vi "rsscope_core_global.vi"() -> ()   [LabVIEW 2014] (continued)
WfmDDNSpectrum1, WfmPNSpectrum1, WfmRNSpectrum1, WfmNBathtub2, WfmNBathMeas2, WfmTNHist2, WfmDNHist2, WfmDDNHist2, WfmPNHist2, WfmRNOHist2, WfmTNTrack2, WfmDDNTrack2, WfmPNTrack2, WfmRNTrack2, WfmTNSpectrum2, WfmDDNSpectrum2, WfmPNSpectrum2, WfmRNSpectrum2, WfmPJDHist1, WfmBUJHist1, WfmRJHist1, WfmPJDTrack1, WfmPJDSpectrum1, WfmPJDHist2, WfmBUJHist2, WfmRJHist2, WfmPJDTrack2, WfmPJDSpectrum2, WfmPNDHist1, WfmBUNHist1, WfmRNHist1, WfmPNDTrack1, WfmPNDSpectrum1, WfmPNDHist2, WfmBUNHist2, WfmRNHist2, WfmPNDTrack2, WfmPNDSpectrum2\r\n\nRemote-control command(s):\nREFLevel<m>:RELative:HYSTeresis"}, {"Level"=2, "Class Only"=TRUE, "Identifier"="", "Descriptive Name"="Tube", "Data Type"=0, "Command"="", "Access"=0, "Range Table"="", "Read Callback"="", "Write Callback"="", "Supported Models"="", "Instrument Options"="", "Flags"=0, "Help"="Configures tube settings for reference levels."}, {"Level"=3, "Class Only"=FALSE, "Identifier"="RSSCOPE_ATTR_TUBE_RELATIVE_OUTER_DISTANCE", "Descriptive Name"="Tube Relative Outer Distance", "Data Type"=1, "Command"="REFL{WfmSuffix}:REL:OTUB", "Access"=2, "Range Table"="RsScope_rngPercent", "Read Callback"="", "Write Callback"="", "Supported Models"="", "Instrument Options"="", "Flags"=0, "Help"="Defines a percentage of the signal level by which the absolute signal level may be larger than the high signal level or lower than the low signal level to be considered high or low, respectively.\n\nAvailable Repeated Capabilities:\nWfmSuffix: WfmNone, WfmC1W1, WfmC1W2, WfmC1W3, WfmC2W1, WfmC2W2, WfmC2W3, WfmC3W1, WfmC3W2, WfmC3W3, WfmC4W1, WfmC4W2, WfmC4W3, WfmMath1, WfmMath2, WfmMath3, WfmMath4, WfmRef1, WfmRef2, WfmRef3, WfmRef4, WfmXY1, WfmXY2, WfmXY3, WfmXY4, WfmMeas1, WfmMeas2, WfmMeas3, WfmMeas4, WfmMeas5, WfmMeas6, WfmMeas7, WfmMeas8, WfmSbus1, WfmSbus2, WfmSbus3, WfmSbus4, WfmD0, WfmD1, WfmD2, WfmD3, WfmD4, WfmD5, WfmD6, WfmD7, WfmD8, WfmD9, WfmD10, WfmD11, WfmD12, WfmD13, WfmD14, WfmD15, WfmMSO1, WfmMSO2, WfmMSO3, WfmMSO4, WfmTRK1, WfmTRK2, WfmTRK3, WfmTRK4, WfmTRK5, WfmTRK6, WfmTRK7, WfmTRK8, WfmSpectrum1, WfmSpectrum2, WfmSpectrum3, WfmSpectrum4, WfmSG1TL1, WfmSG1TL2, WfmSG2TL1, WfmSG2TL2, WfmSG3TL1, WfmSG3TL2, WfmSG4TL1, WfmSG4TL2, WfmEye1, WfmEye2, WfmEye3, WfmEye4, WfmZ1V1, WfmZ1V2, WfmZ1V3, WfmZ1V4, WfmZ1I1, WfmZ1I2, WfmZ1I3, WfmZ1I4, WfmZ2V1, WfmZ2V2, WfmZ2V3, WfmZ2V4, WfmZ2I1, WfmZ2I2, WfmZ2I3, WfmZ2I4, WfmDiff1, WfmDiff2, WfmCommon1, WfmCommon2, WfmTDRZ, WfmTDRH, WfmTDRR, WfmMath5, WfmMath6, WfmMath7, WfmMath8, WfmSpectrum5, WfmSpectrum6, WfmSpectrum7, WfmSpectrum8, WfmSG5TL1, WfmSG5TL2, WfmSG6TL1, WfmSG6TL2, WfmSG7TL1, WfmSG7TL2, WfmSG8TL1, WfmSG8TL2, WfmHP1, WfmHP2, WfmHP3, WfmHP4, WfmHP5, WfmHP6, WfmHP7, WfmHP8, WfmHP9, WfmHP10, WfmBathtub1, WfmBathMeas1, WfmStepResp1, WfmSRHist1, WfmSDHist1, WfmTJHist1, WfmDJHist1, WfmDDJHist1, WfmPJHist1, WfmRJOHist1, WfmSRTrack1, WfmTJTrack1, WfmDJTrack1, WfmDDJTrack1, WfmPJTrack1, WfmRJTrack1, WfmTJSpectrum1, WfmDDJSpectrum1, WfmPJSpectrum1, WfmRJSpectrum1, WfmSEye1, WfmBathtub2, WfmBathMeas2, WfmStepResp2, WfmSRHist2, WfmSDHist2, WfmTJHist2, WfmDJHist2, WfmDDJHist2, WfmPJHist2, WfmRJOHist2, WfmSRTrack2, WfmSDTrack2, WfmTJTrack2, WfmDDJTrack2, WfmPJTrack2, WfmRJTrack2, WfmTJSpectrum2, WfmDDJSpectrum2, WfmPJSpectrum2, WfmRJSpectrum2, WfmSEye2, WfmNBathtub1, WfmNBathMeas1, WfmTNHist1, WfmDNHist1, WfmDDNHist1, WfmPNHist1, WfmRNOTrack1, WfmTNTrack1, WfmDDNTrack1, WfmPNTrack1, WfmRNTrack1, WfmTNSpectrum1, WfmDDNSpectrum1, WfmPNSpectrum1, WfmRNSpectrum1, WfmNBathtub2, WfmNBathMeas2, WfmTNHist2, WfmDNHist2, WfmDDNHist2, WfmPNHist2, WfmRNOHist2, WfmTNTrack2, WfmDDNTrack2, WfmPNTrack2, WfmRNTrack2, WfmTNSpectrum2, WfmDDNSpectrum2, WfmPNSpectrum2, WfmRNSpectrum2, WfmPJDHist1, WfmBUJHist1, WfmRJHist1, WfmPJDTrack1, WfmPJDSpectrum1, WfmPJDHist2, WfmBUJHist2, WfmRJHist2, WfmPJDTrack2, WfmPJDSpectrum2, WfmPNDHist1, WfmBUNHist1, WfmRNHist1, WfmPNDTrack1, WfmPNDSpectrum1, WfmPNDHist2, WfmBUNHist2, WfmRNHist2, WfmPNDTrack2, WfmPNDSpectrum2\r\n\nRemote-control command(s):\nREFLevel<m>:RELative:OTUBe"}, {"Level"=3, "Class Only"=FALSE, "Identifier"="RSSCOPE_ATTR_TUBE_RELATIVE_INNER_DISTANCE", "Descriptive Name"="Tube Relative Inner Distance", "Data Type"=1, "Command"="REFL{WfmSuffix}:REL:ITUB", "Access"=2, "Range Table"="RsScope_rngTubeRelativeInnerDistance", "Read Callback"="", "Write Callback"="", "Supported Models"="", "Instrument Options"="", "Flags"=0, "Help"="Defines a percentage of the signal level by which the absolute signal level may be higher than the low signal level or lower than the high signal level to be considered low or high, respectively.\n\nAvailable Repeated Capabilities:\nWfmSuffix: WfmNone, WfmC1W1, WfmC1W2, WfmC1W3, WfmC2W1, WfmC2W2, WfmC2W3, WfmC3W1, WfmC3W2, WfmC3W3, WfmC4W1, WfmC4W2, WfmC4W3, WfmMath1, WfmMath2, WfmMath3, WfmMath4, WfmRef1, WfmRef2, WfmRef3, WfmRef4, WfmXY1, WfmXY2, WfmXY3, WfmXY4, WfmMeas1, WfmMeas2, WfmMeas3, WfmMeas4, WfmMeas5, WfmMeas6, WfmMeas7, WfmMeas8, WfmSbus1, WfmSbus2, WfmSbus3, WfmSbus4, WfmD0, WfmD1, WfmD2, WfmD3, WfmD4, WfmD5, WfmD6, WfmD7, WfmD8, WfmD9, WfmD10, WfmD11, WfmD12, WfmD13, WfmD14, WfmD15, WfmMSO1, WfmMSO2, WfmMSO3, WfmMSO4, WfmTRK1, WfmTRK2, WfmTRK3, WfmTRK4, WfmTRK5, WfmTRK6, WfmTRK7, WfmTRK8, WfmSpectrum1, WfmSpectrum2, WfmSpectrum3, WfmSpectrum4, WfmSG1TL1, WfmSG1TL2, WfmSG2TL1, WfmSG2TL2, WfmSG3TL1, WfmSG3TL2, WfmSG4TL1, WfmSG4TL2, WfmEye1, WfmEye2, WfmEye3, WfmEye4, WfmZ1V1, WfmZ1V2, WfmZ1V3, WfmZ1V4, WfmZ1I1, WfmZ1I2, WfmZ1I3, WfmZ1I4, WfmZ2V1, WfmZ2V2, WfmZ2V3, WfmZ2V4, WfmZ2I1, WfmZ2I2, WfmZ2I3, WfmZ2I4, WfmDiff1, WfmDiff2, WfmCommon1, WfmCommon2, WfmTDRZ, WfmTDRH, WfmTDRR, WfmMath5, WfmMath6, WfmMath7, WfmMath8, WfmSpectrum5, WfmSpectrum6, WfmSpectrum7, WfmSpectrum8, WfmSG5TL1, WfmSG5TL2, WfmSG6TL1, WfmSG6TL2, WfmSG7TL1, WfmSG7TL2, WfmSG8TL1, WfmSG8TL2, WfmHP1, WfmHP2, WfmHP3, WfmHP4, WfmHP5, WfmHP6, WfmHP7, WfmHP8, WfmHP9, WfmHP10, WfmBathtub1, WfmBathMeas1, WfmStepResp1, WfmSRHist1, WfmSDHist1, WfmTJHist1, WfmDJHist1, WfmDDJHist1, WfmPJHist1, WfmRJOHist1, WfmSRTrack1, WfmTJTrack1, WfmDJTrack1, WfmDDJTrack1, WfmPJTrack1, WfmRJTrack1, WfmTJSpectrum1, WfmDDJSpectrum1, WfmPJSpectrum1, WfmRJSpectrum1, WfmSEye1, WfmBathtub2, WfmBathMeas2, WfmStepResp2, WfmSRHist2, WfmSDHist2, WfmTJHist2, WfmDJHist2, WfmDDJHist2, WfmPJHist2, WfmRJOHist2, WfmSRTrack2, WfmSDTrack2, WfmTJTrack2, WfmDDJTrack2, WfmPJTrack2, WfmRJTrack2, WfmTJSpectrum2, WfmDDJSpectrum2, WfmPJSpectrum2, WfmRJSpectrum2, WfmSEye2, WfmNBathtub1, WfmNBathMeas1, WfmTNHist1, WfmDNHist1, WfmDDNHist1, WfmPNHist1, WfmRNOTrack1, WfmTNTrack1, WfmDDNTrack1, WfmPNTrack1, WfmRNTrack1, WfmTNSpectrum1, WfmDDNSpectrum1, WfmPNSpectrum1, WfmRNSpectrum1, WfmNBathtub2, WfmNBathMeas2, WfmTNHist2, WfmDNHist2, WfmDDNHist2, WfmPNHist2, WfmRNOHist2, WfmTNTrack2, WfmDDNTrack2, WfmPNTrack2, WfmRNTrack2, WfmTNSpectrum2, WfmDDNSpectrum2, WfmPNSpectrum2, WfmRNSpectrum2, WfmPJDHist1, WfmBUJHist1, WfmRJHist1, WfmPJDTrack1, WfmPJDSpectrum1, WfmPJDHist2, WfmBUJHist2, WfmRJHist2, WfmPJDTrack2, WfmPJDSpectrum2, WfmPNDHist1, WfmBUNHist1, WfmRNHist1, WfmPNDTrack1, WfmPNDSpectrum1, WfmPNDHist2, WfmBUNHist2, WfmRNHist2, WfmPNDTrack2, WfmPNDSpectrum2\r\n\nRemote-control command(s):\nREFLevel<m>:RELative:ITUBe"}, {"Level"=3, "Class Only"=FALSE, "Identifier"="RSSCOPE_ATTR_TUBE_ABSOLUTE_TOP_OUTER_DISTANCE", "Descriptive Name"="Tube Absolute Top Outer Distance", "Data Type"=1, "Command"="REFL{WfmSuffix}:ABS:TOT", "Access"=2, "Range Table"="", "Read Callback"="", "Write Callback"="", "Supported Models"="", "Instrument Options"="", "Flags"=0, "Help"="Defines an area above the high signal level which is still considered to be high level.\n\nAvailable Repeated Capabilities:\nWfmSuffix: WfmNone, WfmC1W1, WfmC1W2, WfmC1W3, WfmC2W1, WfmC2W2, WfmC2W3, WfmC3W1, WfmC3W2, WfmC3W3, WfmC4W1, WfmC4W2, WfmC4W3, WfmMath1, WfmMath2, WfmMath3, WfmMath4, WfmRef1, WfmRef2, WfmRef3, WfmRef4, WfmXY1, WfmXY2, WfmXY3, WfmXY4, WfmMeas1, WfmMeas2, WfmMeas3, WfmMeas4, WfmMeas5, WfmMeas6, WfmMeas7, WfmMeas8, WfmSbus1, WfmSbus2, WfmSbus3, WfmSbus4, WfmD0, WfmD1, WfmD2, WfmD3, WfmD4, WfmD5, WfmD6, WfmD7, WfmD8, WfmD9, WfmD10, WfmD11, WfmD12, WfmD13, WfmD14, WfmD15, WfmMSO1, WfmMSO2, WfmMSO3, WfmMSO4, WfmTRK1, WfmTRK2, WfmTRK3, WfmTRK4, WfmTRK5, WfmTRK6, WfmTRK7, WfmTRK8, WfmSpectrum1, WfmSpectrum2, WfmSpectrum3, WfmSpectrum4, WfmSG1TL1, WfmSG1TL2, WfmSG2TL1, WfmSG2TL2, WfmSG3TL1, WfmSG3TL2, WfmSG4TL1, WfmSG4TL2, WfmEye1, WfmEye2, WfmEye3, WfmEye4, WfmZ1V1, WfmZ1V2, WfmZ1V3, WfmZ1V4, WfmZ1I1, WfmZ1I2, WfmZ1I3, WfmZ1I4, WfmZ2V1, WfmZ2V2, WfmZ2V3, WfmZ2V4, WfmZ2I1, WfmZ2I2, WfmZ2I3, WfmZ2I4, WfmDiff1, WfmDiff2, WfmCommon1, WfmCommon2, WfmTDRZ, WfmTDRH, WfmTDRR, WfmMath5, WfmMath6, WfmMath7, WfmMath8, WfmSpectrum5, WfmSpectrum6, WfmSpectrum7, WfmSpectrum8, WfmSG5TL1, WfmSG5TL2, WfmSG6TL1, WfmSG6TL2, WfmSG7TL1, WfmSG7TL2, WfmSG8TL1, WfmSG8TL2, WfmHP1, WfmHP2, WfmHP3, WfmHP4, WfmHP5, WfmHP6, WfmHP7, WfmHP8, WfmHP9, WfmHP10, WfmBathtub1, WfmBathMeas1, WfmStepResp1, WfmSRHist1, WfmSDHist1, WfmTJHist1, WfmDJHist1, WfmDDJHist1, WfmPJHist1, WfmRJOHist1, WfmSRTrack1, WfmTJTrack1, WfmDJTrack1, WfmDDJTrack1, WfmPJTrack1, WfmRJTrack1, WfmTJSpectrum1, WfmDDJSpectrum1, WfmPJSpectrum1, WfmRJSpectrum1, WfmSEye1, WfmBathtub2, WfmBathMeas2, WfmStepResp2, WfmSRHist2, WfmSDHist2, WfmTJHist2, WfmDJHist2, WfmDDJHist2, WfmPJHist2, WfmRJOHist2, WfmSRTrack2, WfmSDTrack2, WfmTJTrack2, WfmDDJTrack2, WfmPJTrack2, WfmRJTrack2, WfmTJSpectrum2, WfmDDJSpectrum2, WfmPJSpectrum2, WfmRJSpectrum2, WfmSEye2, WfmNBathtub1, WfmNBathMeas1, WfmTNHist1, WfmDNHist1, WfmDDNHist1, WfmPNHist1, WfmRNOTrack1, WfmTNTrack1, WfmDDNTrack1, WfmPNTrack1, WfmRNTrack1, WfmTNSpectrum1, WfmDDNSpectrum1, WfmPNSpectrum1, WfmRNSpectrum1, WfmNBathtub2, WfmNBathMeas2, WfmTNHist2, WfmDNHist2, WfmDDNHist2, WfmPNHist2, WfmRNOHist2, WfmTNTrack2, WfmDDNTrack2, WfmPNTrack2, WfmRNTrack2, WfmTNSpectrum2, WfmDDNSpectrum2, WfmPNSpectrum2, WfmRNSpectrum2, WfmPJDHist1, WfmBUJHist1, WfmRJHist1, WfmPJDTrack1, WfmPJDSpectrum1, WfmPJDHist2, WfmBUJHist2, WfmRJHist2, WfmPJDTrack2, WfmPJDSpectrum2, WfmPNDHist1, WfmBUNHist1, WfmRNHist1, WfmPNDTrack1, WfmPNDSpectrum1, WfmPNDHist2, WfmBUNHist2, WfmRNHist2, WfmPNDTrack2, WfmPNDSpectrum2\r\n\nRemote-control command(s):\nREFLevel<m>:ABSolute:TOTube"}, {"Level"=3, "Class Only"=FALSE, "Identifier"="RSSCOPE_ATTR_TUBE_ABSOLUTE_TOP_INNER_DISTANCE", "Descriptive Name"="Tube Absolute Top Inner Distance", "Data Type"=1, "Command"="REFL{WfmSuffix}:ABS:TIT", "Access"=2, "Range Table"="", "Read Callback"="", "Write Callback"="", "Supported Models"="", "Instrument Options"="", "Flags"=0, "Help"="Defines an area beneath the high signal level which is still considered to be high level.\n\nAvailable Repeated Capabilities:\nWfmSuffix: WfmNone, WfmC1W1, WfmC1W2, WfmC1W3, WfmC2W1, WfmC2W2, WfmC2W3, WfmC3W1, WfmC3W2, WfmC3W3, WfmC4W1, WfmC4W2, WfmC4W3, WfmMath1, WfmMath2, WfmMath3, WfmMath4, WfmRef1, WfmRef2, WfmRef3, WfmRef4, WfmXY1, WfmXY2, WfmXY3, WfmXY4, WfmMeas1, WfmMeas2, WfmMeas3, WfmMeas4, WfmMeas5, WfmMeas6, WfmMeas7, WfmMeas8, WfmSbus1, WfmSbus2, WfmSbus3, WfmSbus4, WfmD0, WfmD1, WfmD2, WfmD3, WfmD4, WfmD5, WfmD6, WfmD7, WfmD8, WfmD9, WfmD10, WfmD11, WfmD12, WfmD13, WfmD14, WfmD15, WfmMSO1, WfmMSO2, WfmMSO3, WfmMSO4, WfmTRK1, WfmTRK2, WfmTRK3, WfmTRK4, WfmTRK5, WfmTRK6, WfmTRK7, WfmTRK8, WfmSpectrum1, WfmSpectrum2, WfmSpectrum3, WfmSpectrum4, WfmSG1TL1, WfmSG1TL2, WfmSG2TL1, WfmSG2TL2, WfmSG3TL1, WfmSG3TL2, WfmSG4TL1, WfmSG4TL2, WfmEye1, WfmEye2, WfmEye3, WfmEye4, WfmZ1V1, WfmZ1V2, WfmZ1V3, WfmZ1V4, WfmZ1I1, WfmZ1I2, WfmZ1I3, WfmZ1I4, WfmZ2V1, WfmZ2V2, WfmZ2V3, WfmZ2V4, WfmZ2I1, WfmZ2I2, WfmZ2I3, WfmZ2I4, WfmDiff1, WfmDiff2, WfmCommon1, WfmCommon2, WfmTDRZ, WfmTDRH, WfmTDRR, WfmMath5, WfmMath6, WfmMath7, WfmMath8, WfmSpectrum5, WfmSpectrum6, WfmSpectrum7, WfmSpectrum8, WfmSG5TL1, WfmSG5TL2, WfmSG6TL1, WfmSG6TL2, WfmSG7TL1, WfmSG7TL2, WfmSG8TL1, WfmSG8TL2, WfmHP1, WfmHP2, WfmHP3, WfmHP4, WfmHP5, WfmHP6, WfmHP7, WfmHP8, WfmHP9, WfmHP10, WfmBathtub1, WfmBathMeas1, WfmStepResp1, WfmSRHist1, WfmSDHist1, WfmTJHist1, WfmDJHist1, WfmDDJHist1, WfmPJHist1, WfmRJOHist1, WfmSRTrack1, WfmTJTrack1, WfmDJTrack1, WfmDDJTrack1, WfmPJTrack1, WfmRJTrack1, WfmTJSpectrum1, WfmDDJSpectrum1, WfmPJSpectrum1, WfmRJSpectrum1, WfmSEye1, WfmBathtub2, WfmBathMeas2, WfmStepResp2, WfmSRHist2, WfmSDHist2, WfmTJHist2, WfmDJHist2, WfmDDJHist2, WfmPJHist2, WfmRJOHist2, WfmSRTrack2, WfmSDTrack2, WfmTJTrack2, WfmDDJTrack2, WfmPJTrack2, WfmRJTrack2, WfmTJSpectrum2, WfmDDJSpectrum2, WfmPJSpectrum2, WfmRJSpectrum2, WfmSEye2, WfmNBathtub1, WfmNBathMeas1, WfmTNHist1, WfmDNHist1, WfmDDNHist1, WfmPNHist1, WfmRNOTrack1, WfmTNTrack1, WfmDDNTrack1, WfmPNTrack1, WfmRNTrack1, WfmTNSpectrum1, WfmDDNSpectrum1, WfmPNSpectrum1, WfmRNSpectrum1, WfmNBathtub2, WfmNBathMeas2, WfmTNHist2, WfmDNHist2, WfmDDNHist2, WfmPNHist2, WfmRNOHist2, WfmTNTrack2, WfmDDNTrack2, WfmPNTrack2, WfmRNTrack2, WfmTNSpectrum2, WfmDDNSpectrum2, WfmPNSpectrum2, WfmRNSpectrum2, WfmPJDHist1, WfmBUJHist1, WfmRJHist1, WfmPJDTrack1, WfmPJDSpectrum1, WfmPJDHist2, WfmBUJHist2, WfmRJHist2, WfmPJDTrack2, WfmPJDSpectrum2, WfmPNDHist1, WfmBUNHist1, WfmRNHist1, WfmPNDTrack1, WfmPNDSpectrum1, WfmPNDHist2, WfmBUNHist2, WfmRNHist2, WfmPNDTrack2, WfmPNDSpectrum2\r\n\nRemote-control command(s):\nREFLevel<m>:ABSolute:TITube"}, {"Level"=3, "Class Only"=FALSE, "Identifier"="RSSCOPE_ATTR_TUBE_ABSOLUTE_BOTTOM_INNER_DISTANCE", "Descriptive Name"="Tube Absolute Bottom Inner Distance", "Data Type"=1, "Command"="REFL{WfmSuffix}:ABS:BIT", "Access"=2, "Range Table"="", "Read Callback"="", "Write Callback"="", "Supported Models"="", "Instrument Options"="", "Flags"=0, "Help"="Defines an area above the low signal level which is still considered to be low level.\n\nAvailable Repeated Capabilities:\nWfmSuffix: WfmNone, WfmC1W1, WfmC1W2, WfmC1W3, WfmC2W1, WfmC2W2, WfmC2W3, WfmC3W1, WfmC3W2, WfmC3W3, WfmC4W1, WfmC4W2, WfmC4W3, WfmMath1, WfmMath2, WfmMath3, WfmMath4, WfmRef1, WfmRef2, WfmRef3, WfmRef4, WfmXY1, WfmXY2, WfmXY3, WfmXY4, WfmMeas1, WfmMeas2, WfmMeas3, WfmMeas4, WfmMeas5, WfmMeas6, WfmMeas7, WfmMeas8, WfmSbus1, WfmSbus2, WfmSbus3, WfmSbus4, WfmD0, WfmD1, WfmD2, WfmD3, WfmD4, WfmD5, WfmD6, WfmD7, WfmD8, WfmD9, WfmD10, WfmD11, WfmD12, WfmD13, WfmD14, WfmD15, WfmMSO1, WfmMSO2, WfmMSO3, WfmMSO4, WfmTRK1, WfmTRK2, WfmTRK3, WfmTRK4, WfmTRK5, WfmTRK6, WfmTRK7, WfmTRK8, WfmSpectrum1, WfmSpectrum2, WfmSpectrum3, WfmSpectrum4, WfmSG1TL1, WfmSG1TL2, WfmSG2TL1, WfmSG2TL2, WfmSG3TL1, WfmSG3TL2, WfmSG4TL1, WfmSG4TL2, WfmEye1, WfmEye2, WfmEye3, WfmEye4, WfmZ1V1, WfmZ1V2, WfmZ1V3, WfmZ1V4, WfmZ1I1, WfmZ1I2, WfmZ1I3, WfmZ1I4, WfmZ2V1, WfmZ2V2, WfmZ2V3, WfmZ2V4, WfmZ2I1, WfmZ2I2, WfmZ2I3, WfmZ2I4, WfmDiff1, WfmDiff2, WfmCommon1, WfmCommon2, WfmTDRZ, WfmTDRH, WfmTDRR, WfmMath5, WfmMath6, WfmMath7, WfmMath8, WfmSpectrum5, WfmSpectrum6, WfmSpectrum7, WfmSpectrum8, WfmSG5TL1, WfmSG5TL2, WfmSG6TL1, WfmSG6TL2, WfmSG7TL1, WfmSG7TL2, WfmSG8TL1, WfmSG8TL2, WfmHP1, WfmHP2, WfmHP3, WfmHP4, WfmHP5, WfmHP6, WfmHP7, WfmHP8, WfmHP9, WfmHP10, WfmBathtub1, WfmBathMeas1, WfmStepResp1, WfmSRHist1, WfmSDHist1, WfmTJHist1, WfmDJHist1, WfmDDJHist1, WfmPJHist1, WfmRJOHist1, WfmSRTrack1, WfmTJTrack1, WfmDJTrack1, WfmDDJTrack1, WfmPJTrack1, WfmRJTrack1, WfmTJSpectrum1, WfmDDJSpectrum1, WfmPJSpectrum1, WfmRJSpectrum1, WfmSEye1, WfmBathtub2, WfmBathMeas2, WfmStepResp2, WfmSRHist2, WfmSDHist2, WfmTJHist2, WfmDJHist2, WfmDDJHist2, WfmPJHist2, WfmRJOHist2, WfmSRTrack2, WfmSDTrack2, WfmTJTrack2, WfmDDJTrack2, WfmPJTrack2, WfmRJTrack2, WfmTJSpectrum2, WfmDDJSpectrum2, WfmPJSpectrum2, WfmRJSpectrum2, WfmSEye2, WfmNBathtub1, WfmNBathMeas1, WfmTNHist1, WfmDNHist1, WfmDDNHist1, WfmPNHist1, WfmRNOTrack1, WfmTNTrack1, WfmDDNTrack1, WfmPNTrack1, WfmRNTrack1, WfmTNSpectrum1, WfmDDNSpectrum1, WfmPNSpectrum1, WfmRNSpectrum1, WfmNBathtub2, WfmNBathMeas2, WfmTNHist2, WfmDNHist2, WfmDDNHist2, WfmPNHist2, WfmRNOHist2, WfmTNTrack2, WfmDDNTrack2, WfmPNTrack2, WfmRNTrack2, WfmTNSpectrum2, WfmDDNSpectrum2, WfmPNSpectrum2, WfmRNSpectrum2, WfmPJDHist1, WfmBUJHist1, WfmRJHist1, WfmPJDTrack1, WfmPJDSpectrum1, WfmPJDHist2, WfmBUJHist2, WfmRJHist2, WfmPJDTrack2, WfmPJDSpectrum2, WfmPNDHist1, WfmBUNHist1, WfmRNHist1, WfmPNDTrack1, WfmPNDSpectrum1, WfmPNDHist2, WfmBUNHist2, WfmRNHist2, WfmPNDTrack2, WfmPNDSpectrum2\r\n\nRemote-control command(s):\nREFLevel<m>:ABSolute:BITube"}, {"Level"=3, "Class Only"=FALSE, "Identifier"="RSSCOPE_ATTR_TUBE_ABSOLUTE_BOTTOM_OUTER_DISTANCE", "Descriptive Name"="Tube Absolute Bottom Outer Distance", "Data Type"=1, "Command"="REFL{WfmSuffix}:ABS:BOT", "Access"=2, "Range Table"="", "Read Callback"="", "Write Callback"="", "Supported Models"="", "Instrument Options"="", "Flags"=0, "Help"="Defines an area beneath the low signal level which is still considered to be low level.\n\nAvailable Repeated Capabilities:\nWfmSuffix: WfmNone, WfmC1W1, WfmC1W2, WfmC1W3, WfmC2W1, WfmC2W2, WfmC2W3, WfmC3W1, WfmC3W2, WfmC3W3, WfmC4W1, WfmC4W2, WfmC4W3, WfmMath1, WfmMath2, WfmMath3, WfmMath4, WfmRef1, WfmRef2, WfmRef3, WfmRef4, WfmXY1, WfmXY2, WfmXY3, WfmXY4, WfmMeas1, WfmMeas2, WfmMeas3, WfmMeas4, WfmMeas5, WfmMeas6, WfmMeas7, WfmMeas8, WfmSbus1, WfmSbus2, WfmSbus3, WfmSbus4, WfmD0, WfmD1, WfmD2, WfmD3, WfmD4, WfmD5, WfmD6, WfmD7, WfmD8, WfmD9, WfmD10, WfmD11, WfmD12, WfmD13, WfmD14, WfmD15, WfmMSO1, WfmMSO2, WfmMSO3, WfmMSO4, WfmTRK1, WfmTRK2, WfmTRK3, WfmTRK4, WfmTRK5, WfmTRK6, WfmTRK7, WfmTRK8, WfmSpectrum1, WfmSpectrum2, WfmSpectrum3, WfmSpectrum4, WfmSG1TL1, WfmSG1TL2, WfmSG2TL1, WfmSG2TL2, WfmSG3TL1, WfmSG3TL2, WfmSG4TL1, WfmSG4TL2, WfmEye1, WfmEye2, WfmEye3, WfmEye4, WfmZ1V1, WfmZ1V2, WfmZ1V3, WfmZ1V4, WfmZ1I1, WfmZ1I2, WfmZ1I3, WfmZ1I4, WfmZ2V1, WfmZ2V2, WfmZ2V3, WfmZ2V4, WfmZ2I1, WfmZ2I2, WfmZ2I3, WfmZ2I4, WfmDiff1, WfmDiff2, WfmCommon1, WfmCommon2, WfmTDRZ, WfmTDRH, WfmTDRR, WfmMath5, WfmMath6, WfmMath7, WfmMath8, WfmSpectrum5, WfmSpectrum6, WfmSpectrum7, WfmSpectrum8, WfmSG5TL1, WfmSG5TL2, WfmSG6TL1, WfmSG6TL2, WfmSG7TL1, WfmSG7TL2, WfmSG8TL1, WfmSG8TL2, WfmHP1, WfmHP2, WfmHP3, WfmHP4, WfmHP5, WfmHP6, WfmHP7, WfmHP8, WfmHP9, WfmHP10, WfmBathtub1, WfmBathMeas1, WfmStepResp1, WfmSRHist1, WfmSDHist1, WfmTJHist1, WfmDJHist1, WfmDDJHist1, WfmPJHist1, WfmRJOHist1, WfmSRTrack1, WfmTJTrack1, WfmDJTrack1, WfmDDJTrack1, WfmPJTrack1, WfmRJTrack1, WfmTJSpectrum1, WfmDDJSpectrum1, WfmPJSpectrum1, WfmRJSpectrum1, WfmSEye1, WfmBathtub2, WfmBathMeas2, WfmStepResp2, WfmSRHist2, WfmSDHist2, WfmTJHist2, WfmDJHist2, WfmDDJHist2, WfmPJHist2, WfmRJOHist2, WfmSRTrack2, WfmSDTrack2, WfmTJTrack2, WfmDDJTrack2, WfmPJTrack2, WfmRJTrack2, WfmTJSpectrum2, WfmDDJSpectrum2, WfmPJSpectrum2, WfmRJSpectrum2, WfmSEye2, WfmNBathtub1, WfmNBathMeas1, WfmTNHist1, WfmDNHist1, WfmDDNHist1, WfmPNHist1, WfmRNOTrack1, WfmTNTrack1, WfmDDNTrack1, WfmPNTrack1, WfmRNTrack1, WfmTNSpectrum1, WfmDDNSpectrum1, WfmPNSpectrum1, WfmRNSpectrum1, WfmNBathtub2, WfmNBathMeas2, WfmTNHist2, WfmDNHist2, WfmDDNHist2, WfmPNHist2, WfmRNOHist2, WfmTNTrack2, WfmDDNTrack2, WfmPNTrack2, WfmRNTrack2, WfmTNSpectrum2, WfmDDNSpectrum2, WfmPNSpectrum2, WfmRNSpectrum2, WfmPJDHist1, WfmBUJHist1, WfmRJHist1, WfmPJDTrack1, WfmPJDSpectrum1, WfmPJDHist2, WfmBUJHist2, WfmRJHist2, WfmPJDTrack2, WfmPJDSpectrum2, WfmPNDHist1, WfmBUNHist1, WfmRNHist1, WfmPNDTrack1, WfmPNDSpectrum1, WfmPNDHist2, WfmBUNHist2, WfmRNHist2, WfmPNDTrack2, WfmPNDSpectrum2\r\n\nRemote-control command(s):\nREFLevel<m>:ABSolute:BOTube"}, {"Level"=1, "Class Only"=TRUE, "Identifier"="", "Descriptive Name"="Mathematics", "Data Type"=0, "Command"="", "Access"=0, "Range Table"="", "Read Callback"="", "Write Callback"="", "Supported Models"="", "Instrument Options"="", "Flags"=0, "Help"="The R&S RTO provides different methods of creating mathematical waveforms:\n- Applying mathematical functions to source data\n- Performing FFT analysis on source data"}, {"Level"=2, "Class Only"=TRUE, "Identifier"="", "Descriptive Name"="General Mathematics", "Data Type"=0, "Command"="", "Access"=0, "Range Table"="", "Read Callback"="", "Write Callback"="", "Supported Models"="", "Instrument Options"="", "Flags"=0, "Help"="General mathematics parameters."}, {"Level"=3, "Class Only"=FALSE, "Identifier"="RSSCOPE_ATTR_MATH_WAVEFORM_ENABLED", "Descriptive Name"="Math Waveform Enabled", "Data Type"=3, "Command"="CALC:MATH{Math}:STAT", "Access"=2, "Range Table"="", "Read Callback"="", "Write Callback"="", "Supported Models"="", "Instrument Options"="", "Flags"=0, "Help"="Enables the math waveform display.\n\nAvailable Repeated Capabilities:\nMath: M1, M2, M3, M4, M5, M6, M7, M8\r\n\nRemote-control command(s):\nCALCulate:MATH<m>:STATe"}, {"Level"=3, "Class Only"=FALSE, "Identifier"="RSSCOPE_ATTR_MATH_WAVEFORM_ENVELOPE_SELECTION", "Descriptive Name"="Math Envelope Selection", "Data Type"=0, "Command"="CALC:MATH{Math}:ENVS", "Access"=2, "Range Table"="rsscope_rngWaveformSelection", "Read Callback"="", "Write Callback"="", "Supported Models"="", "Instrument Options"="", "Flags"=0, "Help"="Selects the upper or lower part of the waveform for mathematic calculation, or a combination of both.\n\nThe setting is relevant for waveforms with waveform arithmetic mode &apos;Envelope&apos; or with &apos;Peak detect&apos; decimation. All mathematic operations - except for derivation - can be applied to envelope waveforms and waveforms with &apos;Peak detect&apos; decimation.\n\nAvailable Repeated Capabilities:\nMath: M1, M2, M3, M4, M5, M6, M7, M8\r\n\nRemote-control command(s):\nCALCulate:MATH<m>:ENVSelection"}, {"Level"=3, "Class Only"=FALSE, "Identifier"="RSSCOPE_ATTR_MATH_ACQUISITION_TYPE", "Descriptive Name"="Math Acquisition Type", "Data Type"=0, "Command"="CALC:MATH{Math}:ARIT", "Access"=2, "Range Table"="rsscope_rngWaveformArithmetics", "Read Callback"="", "Write Callback"="", "Supported Models"="", "Instrument Options"="", "Flags"=0, "Help"="Selects the method to build the resulting math waveform from consecutive acquisitions. The processing is similar to the waveform arithmetics - instead of the acquired waveforms the math waveforms are used to create envelope and average.\n\nAvailable Repeated Capabilities:\nMath: M1, M2, M3, M4, M5, M6, M7, M8\r\n\nRemote-control command(s):\nCALCulate:MATH<m>:ARIThmetics"}, {"Level"=3, "Class Only"=FALSE, "Identifier"="RSSCOPE_ATTR_MATH_EXPRESSION", "Descriptive Name"="Math Expression", "Data Type"=2, "Command"="CALC:MATH{Math}", "Access"=2, "Range Table"="", "Read Callback"="", "Write Callback"="", "Supported Models"="", "Instrument Options"="", "Flags"=0, "Help"="Defines the math expression to be calculated for the specified math channel.\n\nAvailable Repeated Capabilities:\nMath: M1, M2, M3, M4, M5, M6, M7, M8\r\n\nRemote-control command(s):\nCALCulate:MATH<m>[:EXPRession][:DEFine]"}, {"Level"=3, "Class Only"=FALSE, "Identifier"="RSSCOPE_ATTR_MATH_VERTICAL_RANGE", "Descriptive Name"="Math Vertical Range", "Data Type"=1, "Command"="CALC:MATH{Math}:VERT:RANG", "Access"=2, "Range Table"="RsScope_rngMathVerticalRange", "Read Callback"="", "Write Callback"="", "Supported Models"="", "Instrument Options"="", "Flags"=0, "Help"="Defines the range of FFT values to be displayed.\n\nAvailable Repeated Capabilities:\nMath: M1, M2, M3, M4, M5, M6, M7, M8\r\n\nRemote-control command(s):\nCALCulate:MATH<m>:VERTical:RANGe"}, {"Level"=3, "Class Only"=FALSE, "Identifier"="RSSCOPE_ATTR_MATH_VERTICAL_SCALE", "Descriptive Name"="Math Vertical Scale", "Data Type"=1, "Command"="CALC:MATH{Math}:VERT:SCAL", "Access"=2, "Range Table"="rsscope_rngMathVerticalScale", "Read Callback"="", "Write Callback"="", "Supported Models"="", "Instrument Options"="", "Flags"=0, "Help"="Defines the scale of the y-axis in the math function diagram. The value is defined as &apos;V per division&apos;, e.g. 50V/div. In this case, the horizontal grid lines are displayed in intervals of 50 V.\n\nAvailable Repeated Capabilities:\nMath: M1, M2, M3, M4, M5, M6, M7, M8\r\n\nRemote-control command(s):\nCALCulate:MATH<m>:VERTical:SCALe"}, {"Level"=3, "Class Only"=FALSE, "Identifier"="RSSCOPE_ATTR_MATH_VERTICAL_OFFSET", "Descriptive Name"="Math Vertical Offset", "Data Type"=1, "Command"="CALC:MATH{Math}:VERT:OFFS", "Access"=2, "Range Table"="RsScope_rngMathVerticalOffset", "Read Callback"="", "Write Callback"="", "Supported Models"="", "Instrument Options"="", "Flags"=0, "Help"="Sets a voltage offset to adjust the vertical position of the math function on the screen.\n\nAvailable Repeated Capabilities:\nMath: M1, M2, M3, M4, M5, M6, M7, M8\r\n\nRemote-control command(s):\nCALCulate:MATH<m>:VERTical:OFFSet"}, {"Level"=3, "Class Only"=FALSE, "Identifier"="RSSCOPE_ATTR_MATH_RESET", "Descriptive Name"="Math Reset", "Data Type"=4, "Command"="ACQ:ARES:IMM", "Access"=1, "Range Table"="", "Read Callback"="", "Write Callback"="", "Supported Models"="", "Instrument Options"="", "Flags"=0, "Help"="Forces the immediate restart of the envelope and average calculation for all waveforms.\n\nAvailable Repeated Capabilities:\nNone\n\nRemote-control command(s):\nACQuire:ARESet:IMMediate"}, {"Level"=3, "Class Only"=FALSE, "Identifier"="RSSCOPE_ATTR_MATH_RESET_MODE", "Descriptive Name"="Math Reset Mode", "Data Type"=0, "Command"="ACQ:ARES:MODE", "Access"=2, "Range Table"="rsscope_rngMathResetMode", "Read Callback"="", "Write Callback"="", "Supported Models"="", "Instrument Options"="", "Flags"=0, "Help"="Defines when the envelope and average evaluation restarts.\n\nAvailable Repeated Capabilities:\nNone\n\nRemote-control command(s):\nACQuire:ARESet:MODE"}, {"Level"=3, "Class Only"=FALSE, "Identifier"="RSSCOPE_ATTR_MATH_ENVELOPE_TIMEOUT", "Descriptive Name"="Math Envelope Timeout", "Data Type"=1, "Command"="ACQ:ARES:TIME", "Access"=2, "Range Table"="rsscope_rngMathEnvelopeTime", "Read Callback"="", "Write Callback"="", "Supported Models"="", "Instrument Options"="", "Flags"=0, "Help"="Defines the time after which the envelope and average evaluation restarts.\n\nAvailable Repeated Capabilities:\nNone\n\nRemote-control command(s):\nACQuire:ARESet:TIME"}, {"Level"=3, "Class Only"=FALSE, "Identifier"="RSSCOPE_ATTR_MATH_ACQUIRED_WAVEFORMS", "Descriptive Name"="Math Acquired Waveforms", "Data Type"=0, "Command"="ACQ:ARES:COUN", "Access"=2, "Range Table"="rsscope_rngMathAcquiredWaveforms", "Read Callback"="", "Write Callback"="", "Supported Models"="", "Instrument Options"="", "Flags"=0, "Help"="Defines the number of acquired waveforms after which the envelope and average evaluation restarts.\n\nAvailable Repeated Capabilities:\nNone\n\nRemote-control command(s):\nACQuire:ARESet:COUNt"}, {"Level"=2, "Class Only"=TRUE, "Identifier"="", "Descriptive Name"="FFT", "Data Type"=0, "Command"="", "Access"=0, "Range Table"="", "Read Callback"="", "Write Callback"="", "Supported Models"="", "Instrument Options"="", "Flags"=0, "Help"="Attributes for setting FFT parameters. During FFT analysis, a signal in the time domain is  converted to a spectrum of frequencies. A basic FFT waveform can be displayed very quickly. By defining additional FFT parameters, the waveform can be configured in more detail. As a result, either the magnitude or the phase of the determined frequencies can be displayed, or more complex FFT functions. Analysis can be restricted to an extract of the original time base, and the results display can be restricted to a specified frequency range."}, {"Level"=3, "Class Only"=FALSE, "Identifier"="RSSCOPE_ATTR_FFT_TYPE", "Descriptive Name"="FFT Type", "Data Type"=0, "Command"="CALC:MATH{Math}:FFT:TYPE", "Access"=2, "Range Table"="RsScope_rngFFTType", "Read Callback"="", "Write Callback"="", "Supported Models"="", "Instrument Options"="", "Flags"=0, "Help"="Selects between the magnitude and phase spectrum type.\n\nAvailable Repeated Capabilities:\nMath: M1, M2, M3, M4, M5, M6, M7, M8\r\n\nRemote-control command(s):\nCALCulate:MATH<m>:FFT:TYPE"}, {"Level"=3, "Class Only"=FALSE, "Identifier"="RSSCOPE_ATTR_FFT_FREQUENCY_AXIS", "Descriptive Name"="FFT Frequency Axis", "Data Type"=0, "Command"="CALC:MATH{Math}:FFT:LOGS", "Access"=2, "Range Table"="RsScope_rngLinLog", "Read Callback"="", "Write Callback"="", "Supported Models"="", "Instrument Options"="", "Flags"=0, "Help"="Defines the scaling method for the frequency (x-)axis of the spectrogram.\n\nAvailable Repeated Capabilities:\nMath: M1, M2, M3, M4, M5, M6, M7, M8\r\n\nRemote-control command(s):\nCALCulate:MATH<m>:FFT:LOGScale"}, {"Level"=3, "Class Only"=FALSE, "Identifier"="RSSCOPE_ATTR_FFT_CENTER_FREQUENCY", "Descriptive Name"="FFT Center Frequency", "Data Type"=1, "Command"="CALC:MATH{Math}:FFT:CFR", "Access"=2, "Range Table"="", "Read Callback"="", "Write Callback"="", "Supported Models"="", "Instrument Options"="", "Flags"=0, "Help"="Defines the position of the displayed frequency range, which is (Center - Span/2) to (Center + Span/2).\n\nAvailable Repeated Capabilities:\nMath: M1, M2, M3, M4, M5, M6, M7, M8\r\n\nRemote-control command(s):\nCALCulate:MATH<m>:FFT:CFRequency"}, {"Level"=3, "Class Only"=FALSE, "Identifier"="RSSCOPE_ATTR_FFT_FREQUENCY_SPAN", "Descriptive Name"="FFT Frequency Span", "Data Type"=1, "Command"="CALC:MATH{Math}:FFT:SPAN", "Access"=2, "Range Table"="", "Read Callback"="", "Write Callback"="", "Supported Models"="", "Instrument Options"="", "Flags"=0, "Help"="The span is specified in Hertz and defines the width of the displayed frequency range, which is (Center - Span/2) to (Center + Span/2).\n\nAvailable Repeated Capabilities:\nMath: M1, M2, M3, M4, M5, M6, M7, M8\r\n\nRemote-control command(s):\nCALCulate:MATH<m>:FFT:SPAN"}, {"Level"=3, "Class Only"=FALSE, "Identifier"="RSSCOPE_ATTR_FFT_FULL_SPAN", "Descriptive Name"="FFT Full Span", "Data Type"=4, "Command"="CALC:MATH{Math}:FFT:FULL", "Access"=1, "Range Table"="", "Read Callback"="", "Write Callback"="", "Supported Models"="", "Instrument Options"="", "Flags"=0, "Help"="Performs FFT calculation for the full frequency span.\n\nAvailable Repeated Capabilities:\nMath: M1, M2, M3, M4, M5, M6, M7, M8\r\n\nRemote-control command(s):\nCALCulate:MATH<m>:FFT:FULLspan"}, {"Level"=3, "Class Only"=FALSE, "Identifier"="RSSCOPE_ATTR_FFT_START_FREQUENCY", "Descriptive Name"="FFT Start Frequency", "Data Type"=1, "Command"="CALC:MATH{Math}:FFT:STAR", "Access"=2, "Range Table"="", "Read Callback"="", "Write Callback"="", "Supported Models"="", "Instrument Options"="", "Flags"=0, "Help"="Defines the start frequency of the displayed frequency span.\n\nAvailable Repeated Capabilities:\nMath: M1, M2, M3, M4, M5, M6, M7, M8\r\n\nRemote-control command(s):\nCALCulate:MATH<m>:FFT:STARt"}, {"Level"=3, "Class Only"=FALSE, "Identifier"="RSSCOPE_ATTR_FFT_STOP_FREQUENCY", "Descriptive Name"="FFT Stop Frequency", "Data Type"=1, "Command"="CALC:MATH{Math}:FFT:STOP", "Access"=2, "Range Table"="", "Read Callback"="", "Write Callback"="", "Supported Models"="", "Instrument Options"="", "Flags"=0, "Help"="Defines the stop frequency of the displayed frequency span.\n\nAvailable Repeated Capabilities:\nMath: M1, M2, M3, M4, M5, M6, M7, M8\r\n\nRemote-control command(s):\nCALCulate:MATH<m>:FFT:STOP"}, {"Level"=3, "Class Only"=FALSE, "Identifier"="RSSCOPE_ATTR_FFT_WINDOW_TYPE", "Descriptive Name"="FFT Window Type", "Data Type"=0, "Command"="CALC:MATH{Math}:FFT:WIND:TYPE", "Access"=2, "Range Table"="rsscope_rngFFTWindowType", "Read Callback"="", "Write Callback"="", "Supported Models"="", "Instrument Options"="", "Flags"=0, "Help"="Windowing helps minimize the discontinuities at the end of the measured signal interval and thus reduces the effect of spectral leakage, increasing the frequency resolution.\nVarious different window functions are provided in the R&S RTO to suit different input signals. Each of the window functions has specific characteristics, including some advantages and some trade-offs. These characteristics need to be considered carefully to find the optimum solution for the measurement task.\n\nAvailable Repeated Capabilities:\nMath: M1, M2, M3, M4, M5, M6, M7, M8\r\n\nRemote-control command(s):\nCALCulate:MATH<m>:FFT:WINDow:TYPE"}, {"Level"=3, "Class Only"=FALSE, "Identifier"="RSSCOPE_ATTR_FFT_USE_COLOR_TABLE", "Descriptive Name"="FFT Use Color Table", "Data Type"=3, "Command"="CALC:MATH{Math}:FFT:USEC", "Access"=2, "Range Table"="", "Read Callback"="", "Write Callback"="", "Supported Models"="", "Instrument Options"="", "Flags"=0, "Help"="If enabled, the selected waveform is displayed according to its assigned color table.\n\nAvailable Repeated Capabilities:\nMath: M1, M2, M3, M4, M5, M6, M7, M8\r\n\nRemote-control command(s):\nCALCulate:MATH<m>:FFT:USEColtab"}, {"Level"=3, "Class Only"=FALSE, "Identifier"="RSSCOPE_ATTR_FFT_REFERENCE_LEVEL", "Descriptive Name"="FFT Reference Level", "Data Type"=1, "Command"="CALC:MATH{Math}:FFT:MAGN:LEV", "Access"=2, "Range Table"="rsscope_rngFFTReferenceLevel", "Read Callback"="", "Write Callback"="", "Supported Models"="", "Instrument Options"="", "Flags"=0, "Help"="Defines the reference level for dB scaling.\n\nAvailable Repeated Capabilities:\nMath: M1, M2, M3, M4, M5, M6, M7, M8\r\n\nRemote-control command(s):\nCALCulate:MATH<m>:FFT:MAGNitude:LEVel"}, {"Level"=3, "Class Only"=FALSE, "Identifier"="RSSCOPE_ATTR_FFT_MAGNITUDE_RANGE", "Descriptive Name"="FFT Magnitude Range", "Data Type"=0, "Command"="CALC:MATH{Math}:FFT:MAGN:RANG", "Access"=2, "Range Table"="rsscope_rngFFTRange", "Read Callback"="", "Write Callback"="", "Supported Models"="", "Instrument Options"="", "Flags"=0, "Help"="Defines the vertical value range in spectrum mode.\n\nAvailable Repeated Capabilities:\nMath: M1, M2, M3, M4, M5, M6, M7, M8\r\n\nRemote-control command(s):\nCALCulate:MATH<m>:FFT:MAGNitude:RANGe"}, {"Level"=3, "Class Only"=FALSE, "Identifier"="RSSCOPE_ATTR_FFT_MAGNITUDE_UNIT", "Descriptive Name"="FFT Magnitude Unit", "Data Type"=0, "Command"="CALC:MATH{Math}:FFT:MAGN:SCAL", "Access"=2, "Range Table"="rsscope_rngFFTMagnitudeUnit", "Read Callback"="", "Write Callback"="", "Supported Models"="", "Instrument Options"="", "Flags"=0, "Help"="Defines the scaling of the y-axis. The display values are valid for 50Ohm termination impendance.\n\nAvailable Repeated Capabilities:\nMath: M1, M2, M3, M4, M5, M6, M7, M8\r\n\nRemote-control command(s):\nCALCulate:MATH<m>:FFT:MAGNitude:SCALe"}, {"Level"=3, "Class Only"=FALSE, "Identifier"="RSSCOPE_ATTR_FFT_PHASE_UNIT", "Descriptive Name"="FFT Phase Unit", "Data Type"=0, "Command"="CALC:MATH{Math}:FFT:PHAS:SCAL", "Access"=2, "Range Table"="rsscope_rngFFTPhaseUnit", "Read Callback"="", "Write Callback"="", "Supported Models"="", "Instrument Options"="", "Flags"=0, "Help"="Defines the scaling unit for phase display.\n\nAvailable Repeated Capabilities:\nMath: M1, M2, M3, M4, M5, M6, M7, M8\r\n\nRemote-control command(s):\nCALCulate:MATH<m>:FFT:PHASe:SCALe"}, {"Level"=3, "Class Only"=FALSE, "Identifier"="RSSCOPE_ATTR_FFT_PHASE_UNWRAP_ENABLED", "Descriptive Name"="FFT Phase Unwrap Enabled", "Data Type"=3, "Command"="CALC:MATH{Math}:FFT:PHAS:UNWR", "Access"=2, "Range Table"="", "Read Callback"="", "Write Callback"="", "Supported Models"="", "Instrument Options"="", "Flags"=0, "Help"="If enabled, phase shifts due to a limitation of the value range are eliminated.\n\nAvailable Repeated Capabilities:\nMath: M1, M2, M3, M4, M5, M6, M7, M8\r\n\nRemote-control command(s):\nCALCulate:MATH<m>:FFT:PHASe:UNWRap"}, {"Level"=3, "Class Only"=FALSE, "Identifier"="RSSCOPE_ATTR_FFT_NOISE_SUPPRESSION_ENABLED", "Descriptive Name"="FFT Noise Suppression Enabled", "Data Type"=3, "Command"="CALC:MATH{Math}:FFT:PHAS:SUPP", "Access"=2, "Range Table"="", "Read Callback"="", "Write Callback"="", "Supported Models"="", "Instrument Options"="", "Flags"=0, "Help"="Enables noise suppression.\n\nAvailable Repeated Capabilities:\nMath: M1, M2, M3, M4, M5, M6, M7, M8\r\n\nRemote-control command(s):\nCALCulate:MATH<m>:FFT:PHASe:SUPPression"}, {"Level"=3, "Class Only"=FALSE, "Identifier"="RSSCOPE_ATTR_FFT_NOISE_SUPPRESSION_THRESHOLD", "Descriptive Name"="FFT Noise Suppression Threshold", "Data Type"=1, "Command"="CALC:MATH{Math}:FFT:PHAS:THR", "Access"=2, "Range Table"="rsscope_rngSuppressionThreshold", "Read Callback"="", "Write Callback"="", "Supported Models"="", "Instrument Options"="", "Flags"=0, "Help"="Defines the minimum frequency magnitude for which phases are calculated.\n\nAvailable Repeated Capabilities:\nMath: M1, M2, M3, M4, M5, M6, M7, M8\r\n\nRemote-control command(s):\nCALCulate:MATH<m>:FFT:PHASe:THReshold"}, {"Level"=3, "Class Only"=FALSE, "Identifier"="RSSCOPE_ATTR_FFT_VERTICAL_MAXIMUM", "Descriptive Name"="FFT Vertical Maximum", "Data Type"=1, "Command"="CALC:MATH{Math}:VERT:MAX", "Access"=2, "Range Table"="RsScope_rngFFTVerticalMaximum", "Read Callback"="", "Write Callback"="", "Supported Models"="", "Instrument Options"="", "Flags"=0, "Help"="Defines the maximum value on y-axis for spectrum displays.\n\nAvailable Repeated Capabilities:\nMath: M1, M2, M3, M4, M5, M6, M7, M8\r\n\nRemote-control command(s):\nCALCulate:MATH<m>:VERTical:MAXimum"}, {"Level"=3, "Class Only"=FALSE, "Identifier"="RSSCOPE_ATTR_FFT_RESOLUTION_BANDWIDTH", "Descriptive Name"="FFT Resolution Bandwidth", "Data Type"=1, "Command"="CALC:MATH{Math}:FFT:BAND", "Access"=2, "Range Table"="rsscope_rngRBW", "Read Callback"="", "Write Callback"="", "Supported Models"="", "Instrument Options"="", "Flags"=0, "Help"="Defines the resolution bandwidth.\n\nAvailable Repeated Capabilities:\nMath: M1, M2, M3, M4, M5, M6, M7, M8\r\n\nRemote-control command(s):\nCALCulate:MATH<m>:FFT:BANDwidth[:RESolution][:VALue]"}, {"Level"=3, "Class Only"=FALSE, "Identifier"="RSSCOPE_ATTR_FFT_RESOLUTION_BANDWIDTH_COUPLING_ENABLED", "Descriptive Name"="FFT Resolution Bandwidth Coupling Enabled", "Data Type"=3, "Command"="CALC:MATH{Math}:FFT:BAND:AUTO", "Access"=2, "Range Table"="", "Read Callback"="", "Write Callback"="", "Supported Models"="", "Instrument Options"="", "Flags"=0, "Help"="Couples the frequency span to the RBW.\n\nAvailable Repeated Capabilities:\nMath: M1, M2, M3, M4, M5, M6, M7, M8\r\n\nRemote-control command(s):\nCALCulate:MATH<m>:FFT:BANDwidth[:RESolution]:AUTO"}, {"Level"=3, "Class Only"=FALSE, "Identifier"="RSSCOPE_ATTR_FFT_RESOLUTION_BANDWIDTH_RATIO", "Descriptive Name"="FFT Resolution Bandwidth Ratio", "Data Type"=0, "Command"="CALC:MATH{Math}:FFT:BAND:RAT", "Access"=2, "Range Table"="rsscope_rngRBWRatio", "Read Callback"="", "Write Callback"="", "Supported Models"="", "Instrument Options"="", "Flags"=0, "Help"="Defines the ratio resolution bandwidth (Hz) / span (Hz).\n\nAvailable Repeated Capabilities:\nMath: M1, M2, M3, M4, M5, M6, M7, M8\r\n\nRemote-control command(s):\nCALCulate:MATH<m>:FFT:BANDwidth[:RESolution]:RATio"}, {"Level"=3, "Class Only"=FALSE, "Identifier"="RSSCOPE_ATTR_FFT_EFFECTIVE_RESOLUTION_BANDWIDTH", "Descriptive Name"="FFT Effective Resolution Bandwidth", "Data Type"=1, "Command"="CALC:MATH{Math}:FFT:BAND:ADJ?", "Access"=0, "Range Table"="", "Read Callback"="", "Write Callback"="", "Supported Models"="", "Instrument Options"="", "Flags"=0, "Help"="Queries the effective resolution bandwidth.\n\nAvailable Repeated Capabilities:\nMath: M1, M2, M3, M4, M5, M6, M7, M8\r\n\nRemote-control command(s):\nCALCulate:MATH<m>:FFT:BANDwidth[:RESolution]:ADJusted?"}, {"Level"=3, "Class Only"=FALSE, "Identifier"="RSSCOPE_ATTR_FFT_RESOLUTION_BANDWIDTH_GATE_COUPLING", "Descriptive Name"="FFT Resolution Bandwidth Gate Coupling", "Data Type"=0, "Command"="CALC:MATH{Math}:FFT:GATE:COUP", "Access"=2, "Range Table"="rsscope_rngRBWGateCoupling", "Read Callback"="", "Write Callback"="", "Supported Models"="", "Instrument Options"="", "Flags"=0, "Help"="Defines the behaviour of the record length or RBW value in dependancy to the other FFT parameters.\n\nAvailable Repeated Capabilities:\nMath: M1, M2, M3, M4, M5, M6, M7, M8\r\n\nRemote-control command(s):\nCALCulate:MATH<m>:FFT:GATE:COUPling"}, {"Level"=3, "Class Only"=FALSE, "Identifier"="RSSCOPE_ATTR_FFT_FRAME_ARITHMETIC", "Descriptive Name"="FFT Frame Arithmetic", "Data Type"=0, "Command"="CALC:MATH{Math}:FFT:FRAM:ARIT", "Access"=2, "Range Table"="rsscope_rngWaveformArithmetics", "Read Callback"="", "Write Callback"="", "Supported Models"="",
